vi "AnimatorExample2.vi"() -> ()   [LabVIEW 2013]
uses:
  Control/AnimatorXControl.xctl
panel:
  out "String":string="Instructions:\n\nThe following animators implement a special right-click menu feature that allows you to configure each animator. Right-click one of the animators and choose Configuration... to display the configuration dialog box. You can specify options, such as animation images and frame rate, for the animator. Animators can work in two modes: Automatic and Use value. Under the Automatic mode, an animator automatically changes the current picture according to the frame rate that you specify. Under the Use value mode, an animator shows a picture according to the frame index value you input.\n\nAn animator has two properties--Frame rate and Reverse. Both properties take effect only when you set an animator to the Automatic mode. If an animator is in the Use value mode, you can set the current frame index by animator value.\n\nThe Animator Project example VI contains two animator XControls. This example sets both animators to the Use value mode. Open the AnimatorProject.lvproj to view the structure of the XControls. Run this VI and try changing the frame index of these animators. Then stop the VI."
  in  "stop":bool
  out "AnimatorXControl":u32(xcontrol)
  in  "Frame index":u32
  # "DSC Module Example Program\nAnimator XControl Example 2"
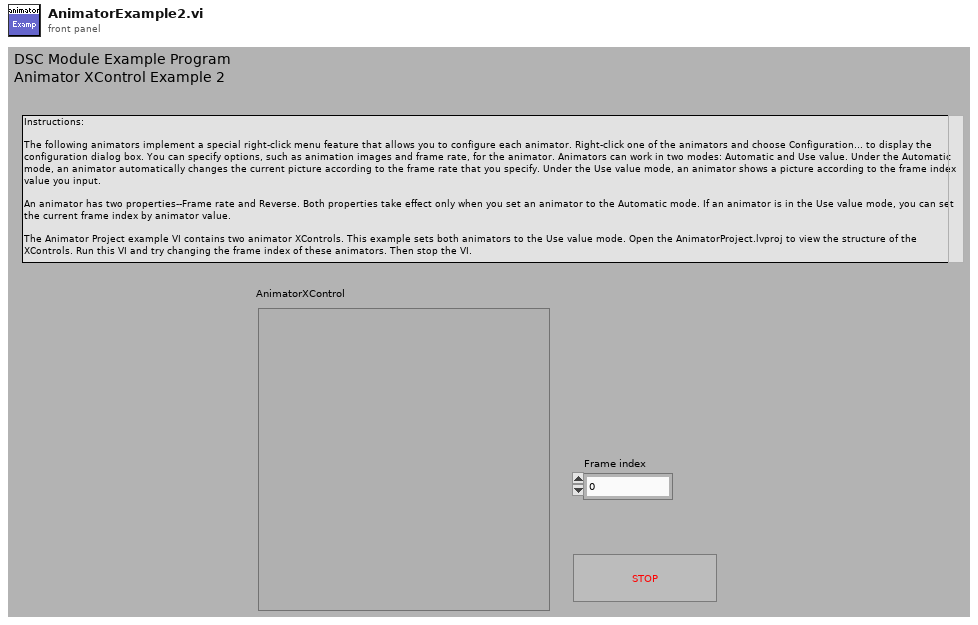
[diagram p1: front panel]
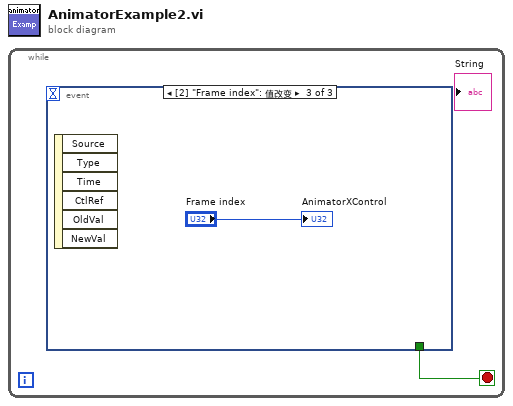
[diagram p0: block diagram]
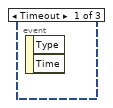
[diagram p2: hidden frame]
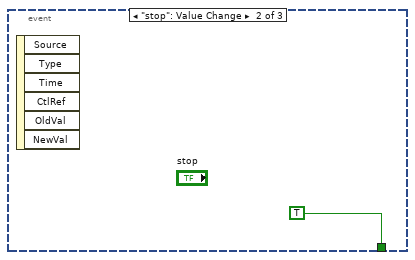
[diagram p3: hidden frame]
diagram:
  n1 = while {
    stop <- w1 stop-if-true
    n2 = event shown="[2] \"Frame index\": 值改变" {
      selector: _ -> [_ _ _]
      dyn-events: _ -> [_ _ _]
      timeout: _ -> [_ _ _]
      tunnel: [_ TRUE _] -> w1
      event Timeout {
        n3 = event-data() -> ()  [unwired: 1 in, 2 out]
      }
      event "stop": Value Change {
        n4 = event-data() -> ()  [unwired: 1 in, 6 out]
      }
      event "Frame index": Value Change {
        n5 = event-data() -> ()  [unwired: 1 in, 6 out]
        "AnimatorXControl" <- "Frame index"
      }
    }
  }
